vi "Get Connection DVR.vi"(8 "error in":errorcluster {"code" format="Error %.0f"}, 11 "NATS Client in":refnum<class "NATS Client.lvclass">) -> (0 "error out":errorcluster {"code" format="Error %.0f"}, 2 "NATS Connection":refnum<data-value>, 3 "NATS Client out":refnum<class "NATS Client.lvclass">)   [LabVIEW 2020, in "NATS Client.lvlib" / "NATS Client.lvclass"]
uses:
  NATS Client.lvclass
  NATS Client.lvclass/NATS Client.ctl
  <vilib>/NATS/NATS Core/Controls/nats connection.ctl
  <vilib>/NATS/NATS Core/NATS Core.lvlib
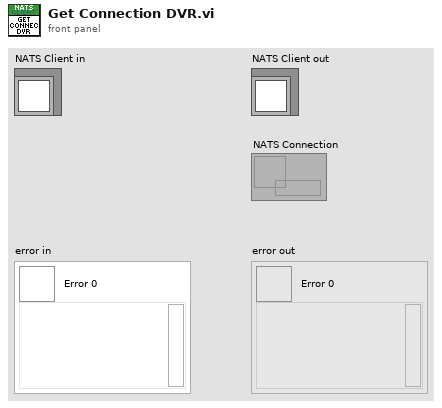
[diagram p1: front panel]
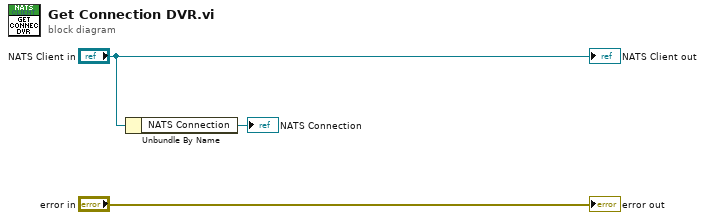
[diagram p0: block diagram]
diagram:
  n1 = Unbundle By Name("NATS Client in") -> ("NATS Connection"=→"NATS Connection":refnum<data-value>)
  "error out" <- "error in"
  "NATS Client out" <- "NATS Client in"
